vi "Handle Modbus.vi"(0 "reference in":refnum<class "Stand.lvclass">, 11 "error in (no error)":errorcluster) -> (4 "reference out":refnum<class "Stand.lvclass">, 14 "Data Read":T1, 15 "error out":errorcluster)   [LabVIEW 2019, in "Stand.lvclass"]
uses:
  Stand.lvclass
  C:/Users/ANENKOV_V1/Desktop/src/Device_class/Device.lvclass
  Modbus_class/ReadData.ctl
  Stand.lvclass/Stand.ctl
  FPGA/TypeDef/AI index.ctl
  AI_class/AI.lvclass/AI.ctl
  AnalogComparator_class/AnalogComparator.lvclass/AnalogComparator.ctl
  Modbus_class/ModbusSp.lvclass/ModbusSp.ctl
  Proccess_class/Proccess.lvclass/Proccess.ctl
  PiecedLinearScale_class/Scale_PiecedLinear.lvclass/Scale_PiecedLinear.ctl
  Logger_class/Logger.lvclass/Logger.ctl
  Modbus_class/ConvertRegToReadData.vi
  Modbus_class/Clear CMD Reg.vi
  PiecedLinearScale_class/RawToScaled.vi
  subvis/Average.vi
  subvis/Loop Time Const.vi
  AI_class/HandleRanges.vi
  AI_class/HandleAlarms.vi
  AI_class/private/WriteToDb.vi
  Proccess_class/GetNames.vi
  Proccess_class/GetLogger.vi
  Modbus_class/ConvertWriteDataToReg.vi
  AnalogComparator_class/GetStatus.vi
  Modbus Data Type Conversation/U16 Array TO SGL Array.vi
  AnalogComparator_class/SetValue.vi
  Logger_class/Enqueue Signal.vi
  Modbus Data Type Conversation/SGL Array to U16 Array.vi
  Modbus Data Type Conversation/SGL to U16.vi
  Device_class/Device.lvclass
  C:/Users/ANENKOV_V1/Desktop/src/Proccess_class/Proccess.lvclass
  AI_class/AI.lvclass
  Logger_class/WriteEvent.vi
  simple_udp/Global - Pressure Data.vi
  <vilib>/gmath/interp.llb/Interpolate 1D.vi
  <vilib>/Utility/error.llb/Error Cluster From Error Code.vi
  AnalogComparator_class/SendToDb.vi
  Modbus_class/STS Cluster to REG.vi
  <vilib>/NI/Modbus Library/API/Slave/Modbus Slave.lvclass
  Modbus_class/ModbusSp.lvclass
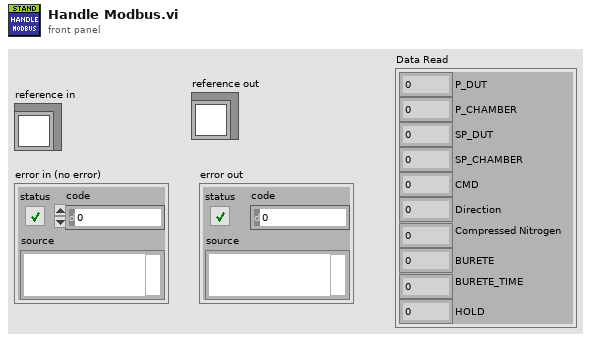
[diagram p1: front panel]
types:
  T1 = typedef "ModbusSp.lvclass/ReadData.ctl" = cluster{"P_DUT":sgl, "P_CHAMBER":sgl, "SP_DUT":sgl, "SP_CHAMBER":sgl, "CMD":u16, "Direction":u16, "Compressed Nitrogen":u16, "BURETE":u16, "BURETE_TIME":u16, "HOLD":u16}
  T2 = typedef "AI index.ctl" = u8
  T3 = typedef "AI_Data.ctl" = cluster{"Stat Data":T4, "OutOfRangeMax":bool, "OutOfRangeMin":bool, "HIHI":bool, "HI":bool, "LO":bool, "LOLO":bool}
  T4 = typedef "AI Statistics Data.ctl" = cluster{"raw mean":dbl, "scl mean":dbl, "raw mean 1Hz":dbl, "scl mean 1Hz":dbl}
  T5 = typedef "Pressure Source.ctl" = enum16{"Internal", "Modbus", "UDP"}
  T6 = typedef "Data.ctl" = cluster{"P_DUT":dbl, "P_Chamber":dbl}
  T7 = typedef "CMD REG.ctl" = cluster{"EXECUTE_SP":bool, "ALARM_PRESS_DOWN_DUT":bool, "ALARM_PRESS_DOWN_CHAMBER":bool, "ALARM_PRESS_DOWN_DUT_CHAMBER":bool, "FILING_DUT":bool, "FILING_CHAMBER":bool, "BLOCK":bool, "PUMP_STATION_OFF":bool, "Leak start":bool, "Leak stop":bool, "Drain":bool}
  T8 = typedef "ModbusSp.lvclass/WriteData.ctl" = cluster{"SP_DUT":sgl, "SP_CHAMBER":sgl, "P_DUT":sgl, "P_CHAMBER":sgl, "STS":u16, "DIR":u16, "Compressed Nitrogen":u16, "ALR":u16, "AI 0":sgl, "AI 1":sgl, "AI 2":sgl, "AI 3":sgl, "AI 4":sgl, "AI 5":sgl, "AI 6":sgl, "AI 7":sgl, "AI 8":sgl, "AI 9":sgl, "AI 10":sgl, "AI 11":sgl, "AI 12":sgl, "STEP":u16}
  T9 = typedef "TCP Slave.lvclass/Connection.ctl" = cluster{"Connected?":bool, "IP address":string, "connection error":errorcluster}
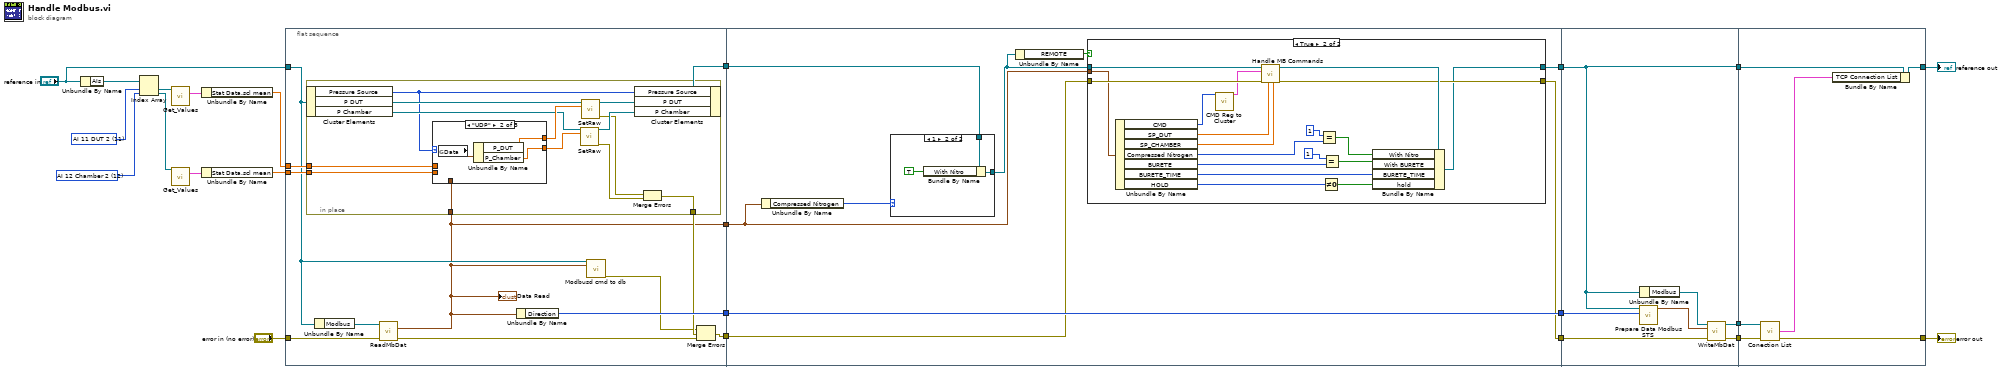
[diagram p0: block diagram]
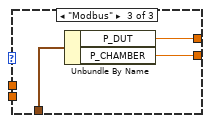
[diagram p3: hidden frame]
diagram:
  w1 = T2 12 items=["AI 0 Cooling Station Level", "AI 1 Cooling Station Temp", "AI 2 Oil Supply Level", "AI 3 Oil Supply Temp", "AI 4 ", "AI 5 Pressure Haskel", "AI 6 Pressure DUT", "AI 7 Pressure Chamber", "AI 8 Pressure Air inlet", "AI 9 Pressure Air outlet", "AI 10 Pressure Messure Line", "AI 11 DUT 2", "AI 12 Chamber 2"] ("AI index")
  w2 = T2 11 items=["AI 0 Cooling Station Level", "AI 1 Cooling Station Temp", "AI 2 Oil Supply Level", "AI 3 Oil Supply Temp", "AI 4 ", "AI 5 Pressure Haskel", "AI 6 Pressure DUT", "AI 7 Pressure Chamber", "AI 8 Pressure Air inlet", "AI 9 Pressure Air outlet", "AI 10 Pressure Messure Line", "AI 11 DUT 2", "AI 12 Chamber 2"] ("AI index")
  n1 = Unbundle By Name("reference in") -> ("AIs"=w9:refnum<class "AI.lvclass">[])
  n2 = Index Array(array=w9, index #1=w2, index #2=w1) -> (element #1=w8:refnum<class "AI.lvclass">, element #2=w5:refnum<class "AI.lvclass">)
  n3 = call "Get_Values.vi"("reference in"=w8) -> ("Data"=w7:T3)  [unwired: 14 in]
  n4 = call "Get_Values.vi"("reference in"=w5) -> ("Data"=w4:T3)  [unwired: 14 in]
  n5 = Unbundle By Name(w7) -> ("Stat Data.scl mean"=w6:dbl)
  n6 = Unbundle By Name(w4) -> ("Stat Data.scl mean"=w3:dbl)
  n7 = flat-sequence {
    tunnel: [w35] -> w17
    tunnel: [w31] -> w15
    tunnel: "reference in" -> [w26]
    tunnel: "error in (no error)" -> [w33]
    tunnel: [w30] -> w13
    tunnel: [w25] -> w11
    tunnel: w6 -> [w28]
    tunnel: w3 -> [w27]
    tunnel: w17 -> [w65]
    tunnel: [w65] -> w16
    tunnel: w15 -> [w58]
    tunnel: [w64] -> w14
    tunnel: w13 -> [w63]
    tunnel: [w62] -> w12
    tunnel: w11 -> [w60]
    tunnel: w16 -> [w96]
    tunnel: w14 -> [w92]
    tunnel: [w92] -> w21
    tunnel: [w95] -> w20
    tunnel: [w94] -> w18
    tunnel: w12 -> [w93]
    tunnel: [w101] -> w22
    tunnel: [w99] -> w19
    tunnel: w21 -> [w103]
    tunnel: w20 -> [w102]
    tunnel: w18 -> [w100]
    frame #0 {
      n8 = Unbundle By Name(w26) -> ("Modbus"=w34:refnum<class "ModbusSp.lvclass">)
      n9 = call "ReadMbDat.vi"("ModbusSp in"=w34, "error in (no error)"=w33) -> ("Data Read"=w25:T1, "error out"=w32:errorcluster)  [unwired: 10 in, 2 out]
      "Data Read" <- w25
      n10 = in-place {
        in-place-border: w25 -> [w46]
        in-place-border: [w39] -> w29
        in-place-border: w28 -> [w37]
        in-place-border: w27 -> [w36]
        n11 = in-place-cluster #1(w26) -> ("Pressure Source"=w38:T5, "P DUT"=w48:refnum<class "AI.lvclass">, "P Chamber"=w44:refnum<class "AI.lvclass">)
        n12 = case shown="\"UDP\"" w38 {
          tunnel: w46 -> [_ _ w56]
          tunnel: [w50 w52 w55] -> w45
          tunnel: [w49 w51 w54] -> w42
          tunnel: w37 -> [w50 _ _]
          tunnel: w36 -> [w49 _ _]
          frame "Internal" {
          }
          frame "UDP" {
            n13 = global read "Global - Pressure Data.vi" "Data"() -> (w53:T6)
            n14 = Unbundle By Name(w53) -> ("P_DUT"=w52:dbl, "P_Chamber"=w51:dbl)
          }
          frame "Modbus" {
            n15 = Unbundle By Name(w56) -> ("P_DUT"=w55:sgl, "P_CHAMBER"=w54:sgl)
          }
        }
        n16 = call "SetRaw.vi"("reference in"=w44, "raw mean"=w42) -> ("reference out"=w43:refnum<class "AI.lvclass">, "error out"=w40:errorcluster)  [unwired: 12 in]
        n17 = call "SetRaw.vi"("reference in"=w48, "raw mean"=w45) -> ("reference out"=w47:refnum<class "AI.lvclass">, "error out"=w41:errorcluster)  [unwired: 12 in]
        n18 = in-place-cluster #1("Pressure Source"=w38, "P DUT"=w47, "P Chamber"=w43) -> (w31:refnum<class "Stand.lvclass">)
        n19 = Merge Errors(w41, w40) -> (w39:errorcluster)
      }
      n20 = Unbundle By Name(w25) -> ("Direction"=w35:u16)
      n21 = call "Modbusd cmd to db.vi"("reference in"=w26, "Data Read"=w25) -> ("error out"=w24:errorcluster)  [unwired: 12 in, 1 out]
      n22 = Merge Errors(w24, w29, w32) -> (w30:errorcluster)
    }
    frame #1 {
      n23 = Unbundle By Name(w60) -> ("Compressed Nitrogen"=w59:u16)
      n24 = case shown="1" w59 {
        tunnel: w58 -> [w66 w69]
        tunnel: [w66 w68] -> w57
        frame Default {
        }
        frame 1 {
          n25 = Bundle By Name(cluster=w69, "With Nitro"=TRUE ("Data.With Nitro")) -> (w68:refnum<class "Stand.lvclass">)
        }
      }
      n26 = Unbundle By Name(w57) -> ("REMOTE"=w61:bool)
      n27 = case shown="True" w61 {
        tunnel: [w71 w81] -> w64
        tunnel: w63 -> [w70 w89]
        tunnel: [w70 w88] -> w62
        tunnel: w60 -> [_ w86]
        tunnel: w57 -> [w71 w87]
        frame False {
        }
        frame True {
          n28 = Unbundle By Name(w86) -> ("CMD"=w85:u16, "SP_DUT"=w83:sgl, "SP_CHAMBER"=w82:sgl, "Compressed Nitrogen"=w79:u16, "BURETE"=w75:u16, "BURETE_TIME"=w80:u16, "HOLD"=w73:u16)
          n29 = call "CMD Reg to Cluster.vi"("CMD Reg"=w85) -> ("CMD REG"=w84:T7)  [unwired: 14 in]
          n30 = call "Handle MB Commands.vi"("SP_CHAMBER"=w82, "SP_DUT"=w83, "error in (no error)"=w89, "CMD REG"=w84, "Stand in"=w87) -> ("error out"=w88:errorcluster, "Stand out"=w90:refnum<class "Stand.lvclass">)  [unwired: 5 in]
          n31 = Equal?(x=u16 1, y=w79) -> (x = y?=w77:bool)
          n32 = Not Equal To 0?(x=w73) -> (x != 0?=w72:bool)
          n33 = Equal?(x=u16 1, y=w75) -> (x = y?=w74:bool)
          n34 = Bundle By Name(cluster=w90, "With Nitro"=w77, "With BURETE"=w74, "BURETE_TIME"=w80, "hold"=w72) -> (w81:refnum<class "Stand.lvclass">)
        }
      }
    }
    frame #2 {
      n35 = call "Prepare Data Modbus STS.vi"("Direction"=w96, "Stand in"=w92) -> ("Data Write"=w97:T8)  [unwired: 9 in]
      n36 = Unbundle By Name(w92) -> ("Modbus"=w91:refnum<class "ModbusSp.lvclass">)
      n37 = call "WriteMbDat.vi"("ModbusSp in"=w91, "Data Write"=w97, "error in (no error)"=w93) -> ("ModbusSp out"=w94:refnum<class "ModbusSp.lvclass">, "error out"=w95:errorcluster)  [unwired: 10 in, 1 out]
    }
    frame #3 {
      n38 = call "Conection List.vi"("ModbusSp in"=w100, "error in (no error)"=w102) -> ("TCP Connection List"=w98:T9[], "error out"=w101:errorcluster)  [unwired: 10 in, 2 out]
      n39 = Bundle By Name(cluster=w103, "TCP Connection List"=w98) -> (w99:refnum<class "Stand.lvclass">)
    }
  }
  "error out" <- w22
  "reference out" <- w19
